vi "Read Type.vi"(8 "error in (no error)":errorcluster, 11 "CSM-Helper in":refnum<class "CSM-Helper.lvclass">) -> (0 "error out":errorcluster, 1 "Part References.Type":T1, 3 "CSM-Helper out":refnum<class "CSM-Helper.lvclass">)   [LabVIEW 2017, in "CSM-Helper.lvclass"]
doc: "### Read Type.vi\n\n-- <b>Controls</b> --\n- <b>CSM-Helper in</b>: CSMHelper input\n\n-- <b>Indicators</b> --\n- <b>Part References.Type</b>:\n- <b>CSM-Helper out</b>: CSMHelper output"
uses:
  CSM-Helper.lvclass
  Utility/CSM Module Type.ctl
  CSM-Helper.lvclass/CSM-Helper.ctl
  Utility/CSM-Helper Utility.lvlib
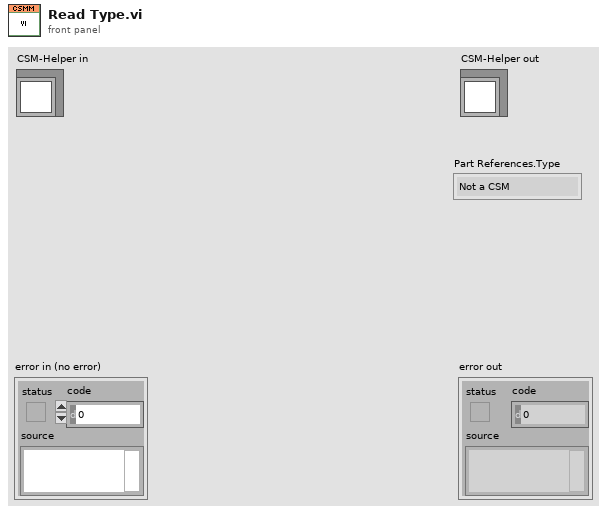
[diagram p1: front panel]
types:
  T1 = typedef "CSM-Helper Utility.lvlib/CSM Module Type.ctl" = enum16{"Not a CSM", "JKISM", "CSM"}
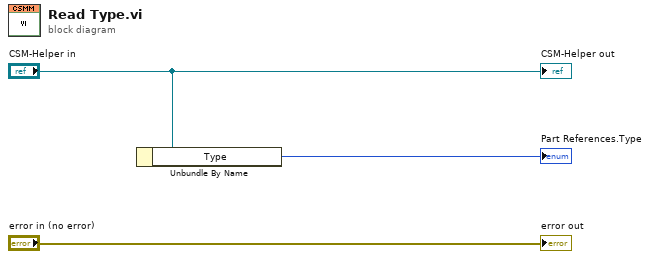
[diagram p0: block diagram]
diagram:
  n1 = Unbundle By Name("CSM-Helper in") -> ("Type"=→"Part References.Type":T1)
  "error out" <- "error in (no error)"
  "CSM-Helper out" <- "CSM-Helper in"
